vi "Auton Edit Queue Order.vi"(10 "Button Cluster":T1, 11 "Boolean":bool) -> ()   [LabVIEW 2016]
uses:
  Common Code/Gamepads/Button Cluster.ctl
  Common Code/Utilities/Change Detect Boolean.vi
  Robot Global Data.vi
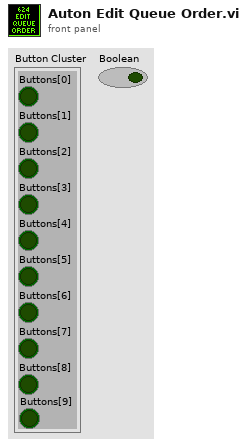
[diagram p1: front panel]
types:
  T1 = typedef "Button Cluster.ctl" = cluster{"Buttons[0]":bool, "Buttons[1]":bool, "Buttons[2]":bool, "Buttons[3]":bool, "Buttons[4]":bool, "Buttons[5]":bool, "Buttons[6]":bool, "Buttons[7]":bool, "Buttons[8]":bool, "Buttons[9]":bool}
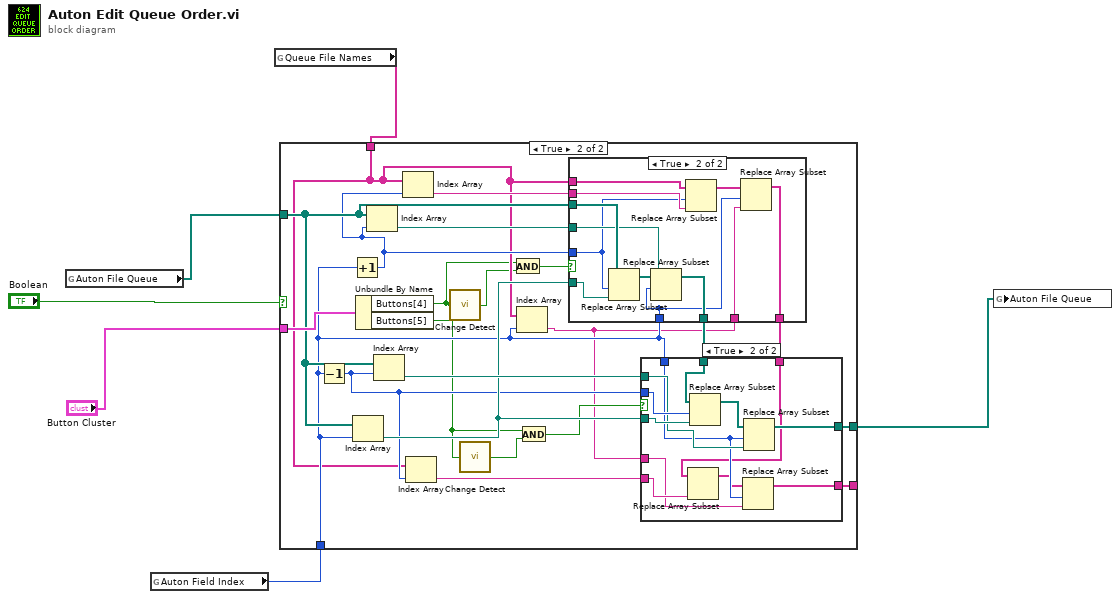
[diagram p0: block diagram]
diagram:
  n1 = global read "Robot Global Data.vi" "Auton File Queue"() -> (w5:path[])
  n2 = global read "Robot Global Data.vi" "Auton Field Index"() -> (w6:i32)
  n3 = global read "Robot Global Data.vi" "Queue File Names"() -> (w4:string[])
  n4 = case shown="True" "Boolean" {
    tunnel: "Button Cluster" -> [_ w30]
    tunnel: w6 -> [_ w17]
    tunnel: w5 -> [w8 w29]
    tunnel: [w8 w24] -> w3
    tunnel: w4 -> [w7 w16]
    tunnel: [w7 w13] -> _
    frame False {
    }
    frame True {
      n5 = Decrement(x=w17) -> (x-1=w20:i32)
      n6 = Increment(x=w17) -> (x+1=w21:i32)
      n7 = Index Array(array=w29, index=w17) -> (element=w26:path)
      n8 = Unbundle By Name(w30) -> ("Buttons[4]"=w10:bool, "Buttons[5]"=w12:bool)
      n9 = Index Array(array=w29, index=w21) -> (element=w28:path)
      n10 = Index Array(array=w29, index=w20) -> (element=w27:path)
      n11 = Index Array(array=w16, index=w21) -> (element=w18:string)
      n12 = Index Array(array=w16, index=w20) -> (element=w19:string)
      n13 = call-poly "Change Detect.vi"("In"=w10) -> ("Changed?"=w9:bool)
      n14 = call-poly "Change Detect.vi"("In"=w12) -> ("Changed?"=w11:bool)
      n15 = And(x=w10, y=w9) -> (x .and. y?=w23:bool)
      n16 = Index Array(array=w16, index=w17) -> (element=w14:string)
      n17 = And(x=w12, y=w11) -> (x .and. y?=w22:bool)
      n18 = case shown="True" w23 {
        tunnel: w29 -> [w46 w58]
        tunnel: w21 -> [_ w48]
        tunnel: w26 -> [_ w57]
        tunnel: w28 -> [_ w55]
        tunnel: w17 -> [_ w47]
        tunnel: [w46 w54] -> w25
        tunnel: w18 -> [_ w52]
        tunnel: w16 -> [w45 w53]
        tunnel: w14 -> [_ w50]
        tunnel: [w45 w49] -> w15
        frame False {
        }
        frame True {
          n19 = Replace Array Subset(array=w58, new element=w57, index=w48) -> (w56:path[])
          n20 = Replace Array Subset(array=w56, new element=w55, index=w47) -> (w54:path[])
          n21 = Replace Array Subset(array=w53, new element=w52, index=w48) -> (w51:string[])
          n22 = Replace Array Subset(array=w51, new element=w50, index=w47) -> (w49:string[])
        }
      }
      n23 = case shown="True" w22 {
        tunnel: w17 -> [_ w38]
        tunnel: w27 -> [_ w40]
        tunnel: w26 -> [_ w43]
        tunnel: w25 -> [w32 w44]
        tunnel: w20 -> [_ w42]
        tunnel: [w32 w39] -> w24
        tunnel: w19 -> [_ w35]
        tunnel: w15 -> [w31 w37]
        tunnel: w14 -> [_ w34]
        tunnel: [w31 w33] -> w13
        frame False {
        }
        frame True {
          n24 = Replace Array Subset(array=w37, new element=w35) -> (w36:string[])  [unwired: 1 in]
          n25 = Replace Array Subset(array=w44, new element=w43, index=w42) -> (w41:path[])
          n26 = Replace Array Subset(array=w36, new element=w34, index=w38) -> (w33:string[])
          n27 = Replace Array Subset(array=w41, new element=w40, index=w38) -> (w39:path[])
        }
      }
    }
  }
  n28 = global write "Robot Global Data.vi" "Auton File Queue"(w3) -> ()
